vi "fo_VerificationSCU.vi"(8 "error in (no error)":errorcluster, 11 "ServerInfo":T1={"port"=107, "AEtitle"="ME", "host"="192.168.10.121", "remoteAE"="DVTK_MW_SCP"}) -> (0 "error out":errorcluster, 2 "status":string, 3 "Succes?":bool)   [LabVIEW 2013, in "main.lvlib"]
uses:
  main.lvlib
  C:/Users/Simon/SkyDrive/LabView/2013/DM2020/bin/Dicom.dll
  bin/Dicom.dll
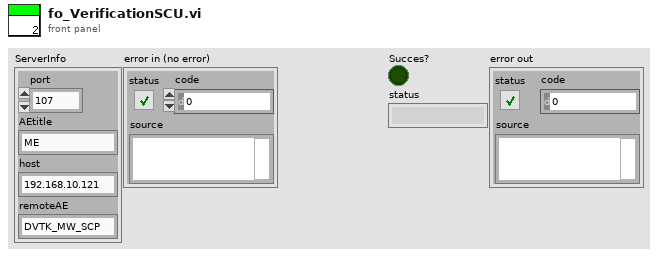
[diagram p1: front panel]
types:
  T1 = cluster{"port":i32, "AEtitle":string, "host":string, "remoteAE":string}
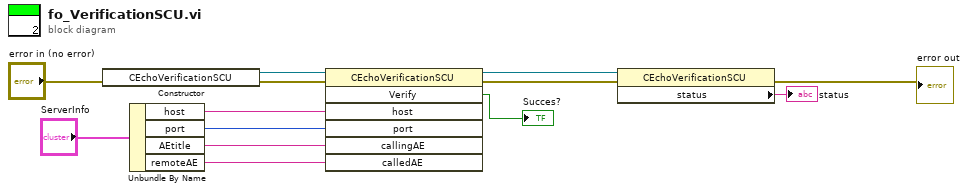
[diagram p0: block diagram]
diagram:
  n1 = constructor class="CEchoVerificationSCU"(error in="error in (no error)") -> (reference out=w12:refnum<k24>, error out=w13:errorcluster)  [unwired: 2 in, 1 out]
  n2 = Unbundle By Name("ServerInfo") -> ("host"=w10:string, "port"=w9:i32, "AEtitle"=w8:string, "remoteAE"=w7:string)
  n3 = invoke class="CEchoVerificationSCU" method="Verify"(reference=w12, error in=w13, "host"=w10, "port"=w9, "callingAE"=w8, "calledAE"=w7) -> (reference out=w6:refnum<k24>, error out=w5:errorcluster, "Verify"=→"Succes?":bool)  [unwired: 1 in, 4 out]
  n4 = property class="CEchoVerificationSCU"(reference=w6, error in=w5) -> (error out=→"error out":errorcluster, "status"=→"status":string)  [unwired: 1 out]
